vi "LIA Substracter.vi"() -> ()   [LabVIEW 2017]
panel:
  out "Numeric Indicator":dbl format="%#_p"
  in  "Min":dbl format="%#_p"
  in  "Max":dbl format="%#_p"
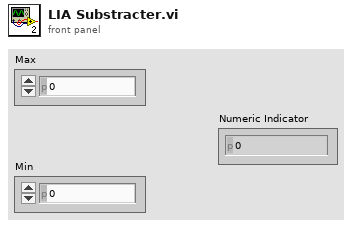
[diagram p1: front panel]
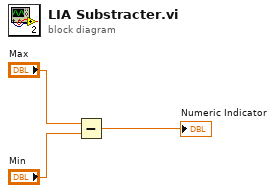
[diagram p0: block diagram]
diagram:
  n1 = Subtract(x="Max", y="Min") -> (x-y=→"Numeric Indicator":dbl)
